vi "Gear Delivery SS Outputs.vi"(11 "Gear Delivery Actuator In":T2={"Gear Release"=enum."Reverse", "Gear Intake"=enum."Off", "Gear Chute"=enum."Off"}) -> (0 "error out":T1)   [LabVIEW 2016]
uses:
  Gear Delivery Actuator Out.ctl
  Gear Delivery Errors.ctl
  Global Variables/Refnum Names.vi
  <vilib>/Rock Robotics/WPI/Solenoid/WPI_SolenoidSetEnum.vi
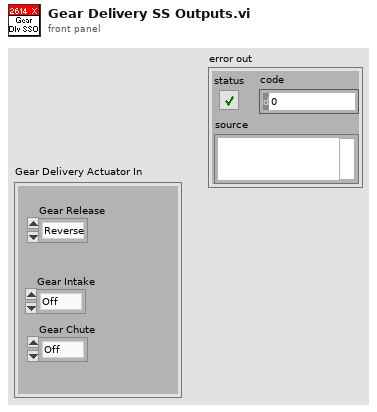
[diagram p1: front panel]
types:
  T1 = typedef "Gear Delivery Errors.ctl" = errorcluster
  T2 = typedef "Gear Delivery Actuator Out.ctl" = cluster{"Gear Release":enum16{"Off", "On", "Forward", "Reverse"}, "Gear Intake":enum16{"Off", "On", "Forward", "Reverse"}, "Gear Chute":enum16{"Off", "On", "Forward", "Reverse"}}
  T3 = typedef "WPI_SolenoidDevRef.ctl" = cluster{"DevStatus":errorcluster, "Pneumatics Control Module":u8, "Forward Solenoid Channel":T4, "Reverse Solenoid Channel":T4}
  T4 = typedef "WPI_SolenoidChannel.ctl" = enum8{"Solenoid 0", "Solenoid 1", "Solenoid 2", "Solenoid 3", "Solenoid 4", "Solenoid 5", "Solenoid 6", "Solenoid 7", "Invalid"}
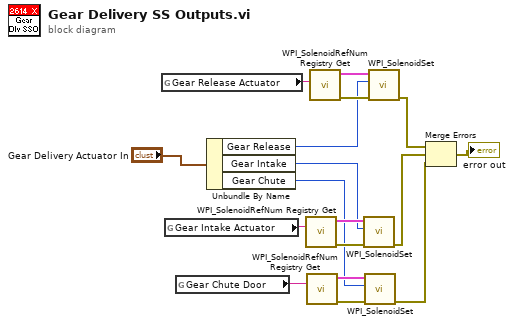
[diagram p0: block diagram]
diagram:
  n1 = global read "Refnum Names.vi" "Gear Release Actuator"() -> (w12:string)
  n2 = global read "Refnum Names.vi" "Gear Intake Actuator"() -> (w11:string)
  n3 = global read "Refnum Names.vi" "Gear Chute Door"() -> (w4:string)
  n4 = Unbundle By Name("Gear Delivery Actuator In") -> ("Gear Release"=w7:enum16{"Off", "On", "Forward", "Reverse"}, "Gear Intake"=w6:enum16{"Off", "On", "Forward", "Reverse"}, "Gear Chute"=w1:enum16{"Off", "On", "Forward", "Reverse"})
  n5 = call <vilib>:"WPI_SolenoidRefNum Registry Get.vi"("refnum name"=w11) -> ("error out"=w16:errorcluster, "SolenoidDevRef"=w15:T3)  [unwired: 9 in]
  n6 = call <vilib>:"WPI_SolenoidRefNum Registry Get.vi"("refnum name"=w4) -> ("error out"=w3:errorcluster, "SolenoidDevRef"=w5:T3)  [unwired: 9 in]
  n7 = call <vilib>:"WPI_SolenoidRefNum Registry Get.vi"("refnum name"=w12) -> ("error out"=w14:errorcluster, "SolenoidDevRef"=w13:T3)  [unwired: 9 in]
  n8 = call-poly <vilib>:"WPI_SolenoidSet.vi"("error in (no error)"=w16, "Value"=w6, "SolenoidDevRef"=w15) -> ("error out"=w9:errorcluster)  [unwired: 7 in, 1 out]
  n9 = call-poly <vilib>:"WPI_SolenoidSet.vi"("error in (no error)"=w3, "Value"=w1, "SolenoidDevRef"=w5) -> ("error out"=w2:errorcluster)  [unwired: 7 in, 1 out]
  n10 = call-poly <vilib>:"WPI_SolenoidSet.vi"("error in (no error)"=w14, "Value"=w7, "SolenoidDevRef"=w13) -> ("error out"=w10:errorcluster)  [unwired: 7 in, 1 out]
  n11 = Merge Errors(w10, w9, w2) -> (→"error out":errorcluster)
